vi "Event Handle Loop_Get Ctl Refnum.vi"(8 "error in (no error)":errorcluster, 11 "QTab Class in":refnum<class "QTab Class.lvclass">) -> (0 "error out":errorcluster, 3 "QTab Class out":refnum<class "QTab Class.lvclass">)   [LabVIEW 2020, in "QTab.lvlib" / "QTab Class.lvclass"]
uses:
  QTab Class.lvclass
  QTab Class.lvclass/QTab Class.ctl
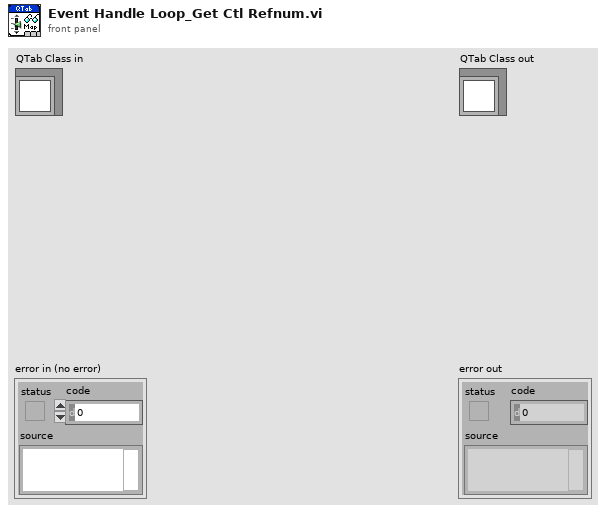
[diagram p1: front panel]
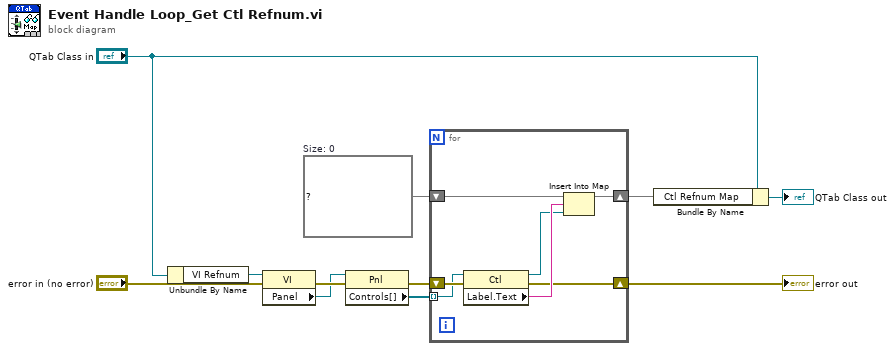
[diagram p0: block diagram]
diagram:
  w9 = map{string, refnum<vi>} {}  # Size: 0
  n1 = Unbundle By Name("QTab Class in") -> ("VI Refnum"=w3:refnum<vi>)
  n2 = property class="VI"(reference=w3, error in="error in (no error)") -> (error out=w11:errorcluster, "Panel"=w10:refnum<vi>)  [unwired: 1 out]
  n3 = property class="Pnl"(reference=w10, error in=w11) -> (error out=w2:errorcluster, "Controls[]"=w1:refnum<vi>[])  [unwired: 1 out]
  n4 = for {
    shift-right: [w13] -> w8
    shift-left: w9 -> [w17]
    shift-right: [w15] -> w6
    shift-left: w2 -> [w18]
    tunnel: w1 -> [w12] mode=indexing
    n5 = property class="Ctl"(reference=w12, error in=w18) -> (reference out=w14:refnum<vi>, error out=w15:errorcluster, "Label.Text"=w16:string)
    n6 = Insert Into Map(map in=w17, key=w16, value=w14) -> (map out=w13:map{string, refnum<vi>})  [unwired: 2 out]
  }
  "error out" <- w6
  n7 = Bundle By Name(cluster="QTab Class in", "Ctl Refnum Map"=w8) -> (→"QTab Class out":refnum<class "QTab Class.lvclass">)
